vi "Display ROIs.vi"(11 "ROI array in":T1[](array[plugin-control])) -> ()   [LabVIEW 2012]
panel:
  out "ROI array":T1[][](array[plugin-control])
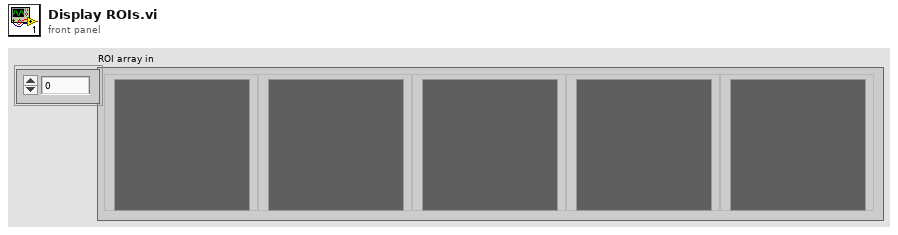
[diagram p1: front panel]
types:
  T1 = typedef "IMAQ Image.ctl" = refnum<image>
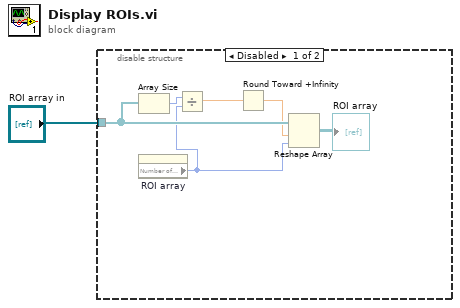
[diagram p0: block diagram]
diagram:
  n1 = disable-structure shown="Disabled" {
    disable-tunnel: "ROI array in" -> [w7 _]
    frame Disabled {
      n2 = Array Size(array=w7) -> (size(s)=w6:i32)
      n3 = property on="ROI array" class="Arr (strict)"() -> ("Number of Columns"=w2:u32)  [unwired: 2 in, 2 out]
      n4 = Divide(x=w6, y=w2) -> (x/y=w5:dbl)
      n5 = Round Toward +Infinity(x=w5) -> (ceil(x): smallest int >= x=w3:dbl)
      n6 = Reshape Array(w7, w3, w2) -> (→"ROI array":T1[][])
    }
    frame Enabled {
    }
  }
